vi "Add Data Channels.vi"(8 "error in (no error)":errorcluster, 9 "progress queue":refnum<queue>, 10 "Framework Configuration":refnum<class "Framework Configuration.lvclass">, 11 "Item Ref in":T1 format="%.0x") -> (0 "error out":errorcluster, 3 "Item Ref out":T1 format="%.0x")   [LabVIEW 2017, in "DSF System Explorer.lvlib"]
uses:
  DSF System Explorer.lvlib
  <vilib>/NI Veristand/Custom Device API/Custom Device Item Ref.ctl
  progress window data.ctl
  DSF Core.lvlibp/Classes/Configuration/Core/Framework/Framework Configuration.lvclass
  Shared/Data Channel Page GUID.vi
  Shared/DSF Shared.lvlib
  <vilib>/NI Veristand/Custom Device API/Custom Device API.lvlib
  DSF Core.lvlibp/Classes/Configuration/Core/Group/Group Configuration.lvclass
  DSF Core.lvlibp/Classes/Configuration/Core/Plugin/Plugin Configuration.lvclass
  DSF Core.lvlibp/Classes/Configuration/Core/Thread/Thread Configuration.lvclass
  DSF Core.lvlibp/Classes/Configuration/Core/Transfer/Transfer Configuration.lvclass
  DSF Core.lvlibp/Classes/Configuration/Core/Core Configuration.lvclass
  C:/Git/DSF/VeriStand/Data Sharing Custom Device/Source/DSF Core.lvlibp/Classes/Configuration/Core/Core Configuration.lvclass
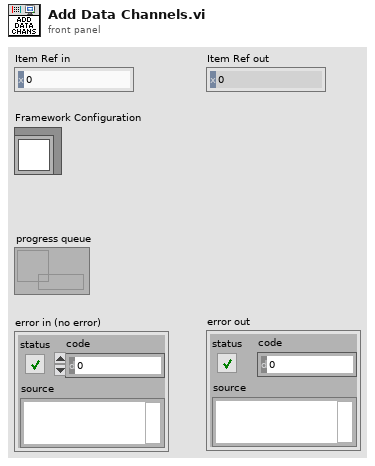
[diagram p1: front panel]
types:
  T1 = typedef "Custom Device API.lvlib/Custom Device Item Ref.ctl" = u64
  T2 = typedef "DSF Core.lvlibp/Plugin Configuration.lvclass/Core Plugin Configuration.ctl" = cluster{"name":string, "components":string[], "cycle timing":T3}
  T3 = typedef "DSF Core.lvlibp/DSF Timing Info.ctl" = cluster{"priority":u64, "decimation":u64, "offset":u64}
  T4 = typedef "DSF Core.lvlibp/DSF Settings Info.ctl" = cluster{"component":string, "values":cluster{"key":string, "value":string}[]}
  T5 = typedef "DSF Core.lvlibp/Thread Configuration.lvclass/Core Thread Configuration.ctl" = cluster{"processor":i32, "priority offset":i16}
  T6 = typedef "DSF Core.lvlibp/Group Configuration.lvclass/Core Group Configuration.ctl" = cluster{"name":string, "direction":T7, "cycle timing":T3, "timeout behavior":T8, "enable conversion":bool}
  T7 = typedef "DSF Core.lvlibp/DSF Direction.ctl" = enum8{"Tx", "Rx"}
  T8 = typedef "DSF Core.lvlibp/DSF Timeout Behavior.ctl" = enum8{"Increment Late Count", "Throw Error"}
  T9 = typedef "DSF Core.lvlibp/Transfer Configuration.lvclass/Core Transfer Configuration.ctl" = cluster{"name":string}
  T10 = typedef "DSF Core.lvlibp/Transfer Configuration.lvclass/Channel Configuration.ctl" = cluster{"configuration":T11, "component settings":T4[]}
  T11 = typedef "DSF Core.lvlibp/Channel Configuration.lvclass/Core Channel Configuration.ctl" = cluster{"name":string, "units":string, "engine data type":T12, "string data type":T12, "string offset":u64}
  T12 = typedef "DSF Core.lvlibp/DSF Data Type.ctl" = enum8{"Bool", "SGL", "DBL", "I8", "I16", "I32", "I64", "U8", "U16", "U32", "U64"}
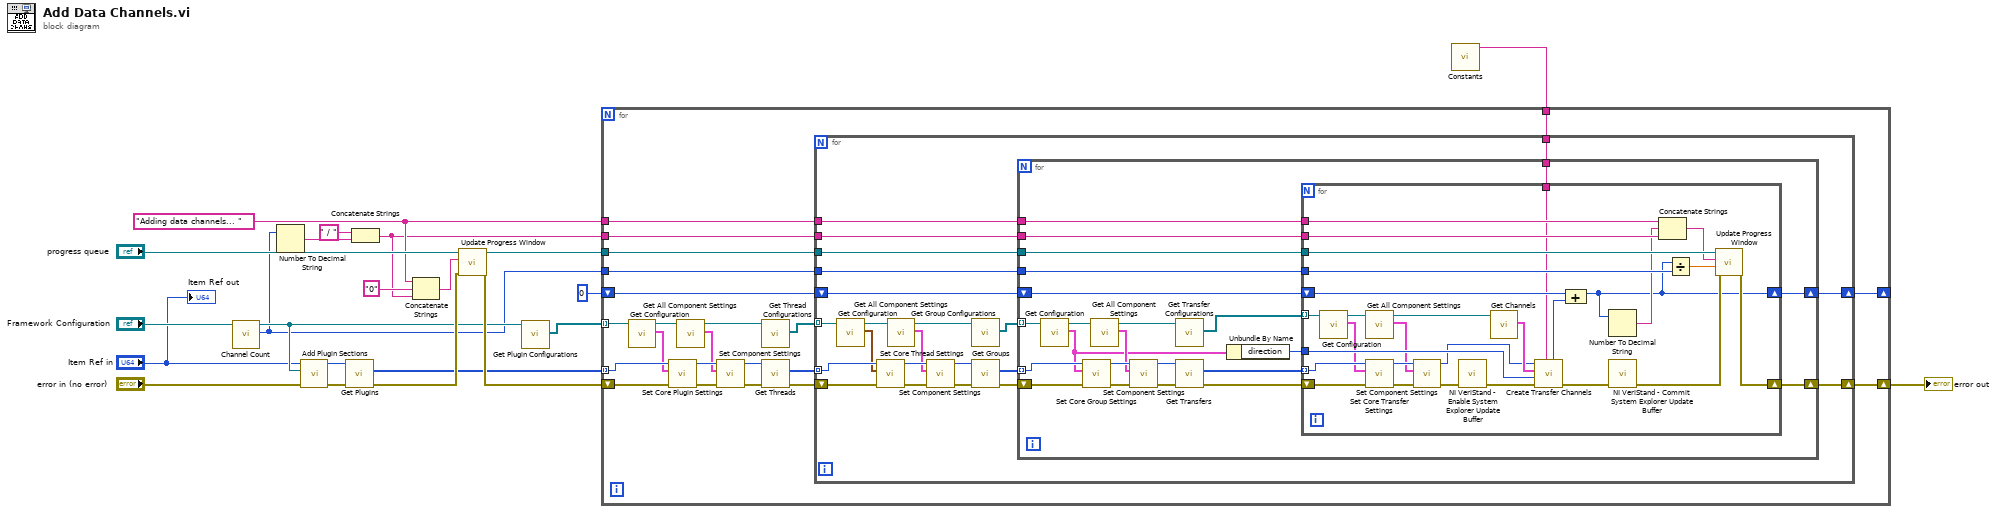
[diagram p0: block diagram]
diagram:
  w13 = "Adding data channels... " ("message (\"\")")
  n1 = call-dynamic "Channel Count.vi"("Framework Configuration in"="Framework Configuration") -> ("channel count"=w3:i32, "Framework Configuration out"=w4:refnum<class "Framework Configuration.lvclass">)  [unwired: 8 in, 1 out]
  n2 = Number To Decimal String(number=w3) -> (decimal integer string=w17:string)  [unwired: 1 in]
  n3 = call "Add Plugin Sections.vi"("error in (no error)"="error in (no error)", "Framework Configuration"=w4, "Item Ref in"="Item Ref in") -> ("error out"=w20:errorcluster, "Item Ref out"=w19:T1)  [unwired: 7 in]
  n4 = call "Get Plugins.vi"("error in (no error)"=w20, "Item Ref in"=w19) -> ("error out"=w10:errorcluster, "Plugin refs"=w9:T1[])  [unwired: 7 in, 1 out]
  n5 = Concatenate Strings(" / " ("string"), w17) -> (w12:string)
  n6 = Concatenate Strings(w13, "0" ("string"), w12) -> (w11:string)
  n7 = call "Update Progress Window.vi"("error in (no error)"=w10, "message (\"\")"=w11, "progress queue in"="progress queue") -> ("error out"=w22:errorcluster, "progress queue out"=w15:refnum<queue>)  [unwired: 7 in]
  n8 = call "Get Plugin Configurations.vi"("Framework Configuration in"=w4) -> ("Plugin Configurations"=w7:refnum<class "Plugin Configuration.lvclass">[])  [unwired: 8 in, 2 out]
  n9 = call-poly "Constants.vi"() -> ("Status GUID"=w8:string)  [unwired: 11 in]
  n10 = for {
    tunnel: w15 -> [w43]
    tunnel: w13 -> [w42]
    tunnel: w12 -> [w41]
    tunnel: w9 -> [w29] mode=indexing
    tunnel: w8 -> [w40]
    tunnel: w3 -> [w39]
    tunnel: w7 -> [w31] mode=indexing
    shift-right: [w44] -> w21
    shift-left: w22 -> [w30]
    shift-right: [w37] -> _
    shift-left: 0 ("channel count") -> [w38]
    n11 = call "Get Configuration.vi"("Core Plugins Configuration in"=w31) -> ("configuration"=w28:T2, "Core Plugins Configuration out"=w25:refnum<class "Plugin Configuration.lvclass">)  [unwired: 8 in, 1 out]
    n12 = call "Set Core Plugin Settings.vi"("error in (no error)"=w30, "plugin configuration"=w28, "Item Ref in"=w29) -> ("error out"=w27:errorcluster, "Item Ref out"=w26:T1)  [unwired: 7 in]
    n13 = call "Get All Component Settings.vi"("Runtime Configuration in"=w25) -> ("component settings"=w24:T4[], "Runtime Configuration out"=w23:refnum<class "Plugin Configuration.lvclass">)  [unwired: 8 in, 1 out]
    n14 = call "Set Component Settings.vi"("error in (no error)"=w27, "component settings"=w24, "Item Ref in"=w26) -> ("error out"=w32:errorcluster, "Item Ref out"=w33:T1)  [unwired: 7 in]
    n15 = call "Get Thread Configurations.vi"("Plugin Configuration in"=w23) -> ("Thread Configurations"=w36:refnum<class "Thread Configuration.lvclass">[])  [unwired: 8 in, 2 out]
    n16 = call "Get Threads.vi"("error in (no error)"=w32, "Item Ref in"=w33) -> ("error out"=w35:errorcluster, "Plugin refs"=w34:T1[])  [unwired: 7 in, 1 out]
    n17 = for {
      tunnel: w34 -> [w53] mode=indexing
      shift-right: [w58] -> w44
      shift-left: w35 -> [w54]
      tunnel: w43 -> [w64]
      tunnel: w41 -> [w63]
      shift-right: [w61] -> w37
      shift-left: w38 -> [w62]
      tunnel: w42 -> [w60]
      tunnel: w39 -> [w59]
      tunnel: w40 -> [w57]
      tunnel: w36 -> [w55] mode=indexing
      n18 = call "Get Configuration.vi"("Core Threads Configuration in"=w55) -> ("configuration"=w51:T5, "Core Threads Configuration out"=w52:refnum<class "Thread Configuration.lvclass">)  [unwired: 8 in, 1 out]
      n19 = call "Set Core Thread Settings.vi"("error in (no error)"=w54, "thread configuration"=w51, "Item Ref in"=w53) -> ("error out"=w50:errorcluster, "Item Ref out"=w49:T1)  [unwired: 7 in]
      n20 = call "Get All Component Settings.vi"("Runtime Configuration in"=w52) -> ("component settings"=w45:T4[], "Runtime Configuration out"=w46:refnum<class "Thread Configuration.lvclass">)  [unwired: 8 in, 1 out]
      n21 = call "Set Component Settings.vi"("error in (no error)"=w50, "component settings"=w45, "Item Ref in"=w49) -> ("error out"=w47:errorcluster, "Item Ref out"=w48:T1)  [unwired: 7 in]
      n22 = call "Get Group Configurations.vi"("Thread Configuration in"=w46) -> ("Group Configurations"=w56:refnum<class "Group Configuration.lvclass">[])  [unwired: 8 in, 2 out]
      n23 = call "Get Groups.vi"("error in (no error)"=w47, "Plugin Ref in"=w48) -> ("error out"=w66:errorcluster, "Group refs"=w65:T1[])  [unwired: 7 in, 1 out]
      n24 = for {
        shift-right: [w81] -> w58
        shift-left: w66 -> [w77]
        tunnel: w65 -> [w76] mode=indexing
        tunnel: w56 -> [w71] mode=indexing
        tunnel: w64 -> [w87]
        tunnel: w63 -> [w85]
        shift-right: [w84] -> w61
        shift-left: w62 -> [w86]
        tunnel: w60 -> [w83]
        tunnel: w59 -> [w82]
        tunnel: w57 -> [w80]
        n25 = call "Get Configuration.vi"("Core Groups Configuration in"=w71) -> ("configuration"=w67:T6, "Core Groups Configuration out"=w70:refnum<class "Group Configuration.lvclass">)  [unwired: 8 in, 1 out]
        n26 = call "Set Core Group Settings.vi"("error in (no error)"=w77, "group configuration"=w67, "Item Ref in"=w76) -> ("error out"=w75:errorcluster, "Item Ref out"=w74:T1)  [unwired: 7 in]
        n27 = call "Get All Component Settings.vi"("Runtime Configuration in"=w70) -> ("component settings"=w69:T4[], "Runtime Configuration out"=w68:refnum<class "Group Configuration.lvclass">)  [unwired: 8 in, 1 out]
        n28 = call "Set Component Settings.vi"("error in (no error)"=w75, "component settings"=w69, "Item Ref in"=w74) -> ("error out"=w73:errorcluster, "Item Ref out"=w72:T1)  [unwired: 7 in]
        n29 = call "Get Transfer Configurations.vi"("Group Configuration in"=w68) -> ("Transfer Configurations"=w79:refnum<class "Transfer Configuration.lvclass">[])  [unwired: 8 in, 2 out]
        n30 = call "Get Transfers.vi"("error in (no error)"=w73, "Group Ref in"=w72) -> ("error out"=w89:errorcluster, "Transfer refs"=w88:T1[])  [unwired: 7 in, 1 out]
        n31 = Unbundle By Name(w67) -> ("direction"=w78:T7)
        n32 = for {
          shift-right: [w112] -> w81
          shift-left: w89 -> [w101]
          tunnel: w88 -> [w99] mode=indexing
          tunnel: w87 -> [w117]
          shift-right: [w104] -> w84
          shift-left: w86 -> [w116]
          tunnel: w85 -> [w113]
          tunnel: w83 -> [w114]
          tunnel: w82 -> [w109]
          tunnel: w78 -> [w98]
          tunnel: w79 -> [w100] mode=indexing
          tunnel: w80 -> [w103]
          n33 = call "Get Configuration.vi"("Core Transfers Configuration in"=w100) -> ("configuration"=w97:T9, "Core Transfers Configuration out"=w92:refnum<class "Transfer Configuration.lvclass">)  [unwired: 8 in, 1 out]
          n34 = call "Get All Component Settings.vi"("Runtime Configuration in"=w92) -> ("component settings"=w91:T4[], "Runtime Configuration out"=w90:refnum<class "Transfer Configuration.lvclass">)  [unwired: 8 in, 1 out]
          n35 = call "Set Core Transfer Settings.vi"("error in (no error)"=w101, "transfer configuration"=w97, "Item Ref in"=w99) -> ("error out"=w96:errorcluster, "Item Ref out"=w95:T1)  [unwired: 7 in]
          n36 = call "Set Component Settings.vi"("error in (no error)"=w96, "component settings"=w91, "Item Ref in"=w95) -> ("error out"=w93:errorcluster, "Item Ref out"=w94:T1)  [unwired: 7 in]
          n37 = call <vilib>:"NI VeriStand - Enable System Explorer Update Buffer.vi"("error in (no error)"=w93) -> ("error out"=w107:errorcluster)  [unwired: 10 in]
          n38 = call "Get Channels.vi"("Transfer Configuration in"=w90) -> ("channels"=w102:T10[])  [unwired: 8 in, 2 out]
          n39 = call "Create Transfer Channels.vi"("GUID (Default Channel)"=w103, "error in (no error)"=w107, "direction"=w98, "channels"=w102, "Item Ref in"=w94) -> ("error out"=w106:errorcluster, "channel count"=w115:i32)  [unwired: 4 in, 1 out]
          n40 = Compound Arithmetic op=ADD(w116, w115) -> (w104:i32)
          n41 = Number To Decimal String(number=w104) -> (decimal integer string=w108:string)  [unwired: 1 in]
          n42 = call <vilib>:"NI VeriStand - Commit System Explorer Update Buffer.vi"("error in (no error)"=w106) -> ("error out"=w105:errorcluster)  [unwired: 10 in]
          n43 = Concatenate Strings(w114, w108, w113) -> (w111:string)
          n44 = Divide(x=w104, y=w109) -> (x/y=w110:dbl)
          n45 = call "Update Progress Window.vi"("error in (no error)"=w105, "progress (0)"=w110, "message (\"\")"=w111, "progress queue in"=w117) -> ("error out"=w112:errorcluster)  [unwired: 6 in, 1 out]
        }
      }
    }
  }
  "error out" <- w21
  "Item Ref out" <- "Item Ref in"
